vi "Set Project Number.vi"(8 "error in (no error)":errorcluster, 10 "Project Number":i32, 11 "Project Number Msg in":refnum<class "Project Number Msg.lvclass">) -> (0 "error out":errorcluster, 3 "Project Number Msg out":refnum<class "Project Number Msg.lvclass">)   [LabVIEW 2013, in "Main Model.lvlib" / "Project Number Msg.lvclass"]
uses:
  Project Number Msg.lvclass
  Project Number Msg.lvclass/Project Number Msg.ctl
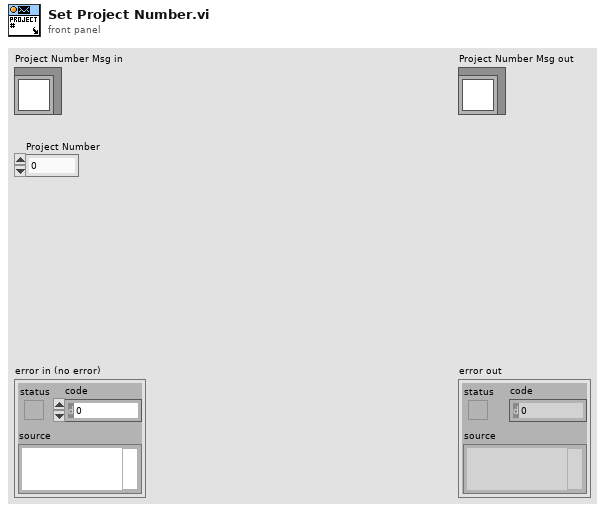
[diagram p1: front panel]
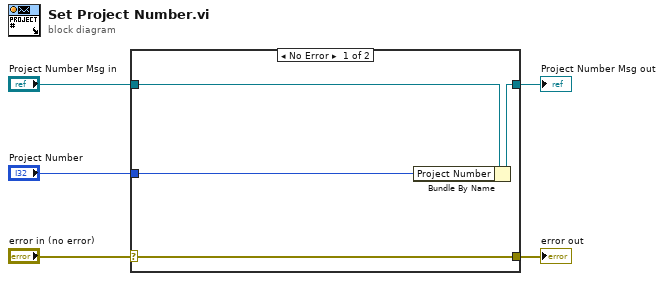
[diagram p0: block diagram]
diagram:
  n1 = case shown="No Error" "error in (no error)" {
    selector: "error in (no error)" -> [w9 w10]
    tunnel: [w9 w10] -> w4
    tunnel: [w7 w11] -> w2
    tunnel: "Project Number Msg in" -> [w8 w11]
    tunnel: "Project Number" -> [w6 _]
    frame No Error {
      n2 = Bundle By Name(cluster=w8, "Project Number"=w6) -> (w7:refnum<class "Project Number Msg.lvclass">)
    }
    frame Error {
    }
  }
  "error out" <- w4
  "Project Number Msg out" <- w2
